vi "generateBarPosAreaCirc.vi"(7 "Number of Denfenders\nWhithout Duelist":i32, 8 "error in (no error)":errorcluster, 9 "AI Parameters":T1={"GotoKick"={"Dist do cone a frente"=150.0, "attacker farback"=1500.0, "Perto"=300.0, "min dist to kick"=150.0, "kick eps"=0.0, "Time to transition"=0.05}, "Attacker"={"CC chute"=0.09, "CC passe"=0.045, "Kick Force"=100.0, "ball-robot Kick"=200.0, "ball-robot Pass"=0.3, "drible\nAttk"=FALSE}, "Defender"={"D max"=1700.0, "Vel p/ robô av"=1000.0, "Kick Force"=100.0, "D atk-def"=0.0, "D farback"=0.0, "drible\ndef"=FALSE, "drible\ngoalie"=FALSE}, "Timeout"={"Field/v in x"=6.0, "Dist Robots"=300, "Dist up in y"=300}, "Pose Striker"={"dist"=200.0, "Numeric"=-4.0, "dist 2"=200.0, "drible\nstriker"=FALSE}, "Dist Stop"=300.0, "D ball out"=200, "D central gap "=150.0, "T pass"=0.0, "Force ++"=0.0, "range kick"=0.0, "Chute alto"=TRUE, "Marcador novo"=TRUE, "drible"=FALSE, "D drible"=300.0, "Versão Striker"=enum."Auto", "Defesa"=enum."ManMark", "Marcador"=enum."Marcar Segundo mais perigoso", "Receptor passe"=enum."Auto", "Área"=enum."Quadrada", "Decisão\nsimples?"=FALSE} {"D drible" format="%#_13g"; "D central gap" format="%#_13g"; "Dist Stop" format="%#_13g"; "Pose Striker"."Numeric" format="%#_13g"; "Defender"."Kick Force" format="%#_13g"; "Defender"."Vel p/ robô av" format="%#_13g"; "Attacker"."ball-robot Kick" format="%#_13g"; "Attacker"."Kick Force" format="%#_13g"; "Attacker"."CC passe" format="%#_13g"; "Attacker"."CC chute" format="%#_13g"; "GotoKick"."kick eps" format="%#_13g"; "GotoKick"."min dist to kick" format="%#_13g"; "GotoKick"."Perto" format="%#_13g"; "GotoKick"."attacker farback" format="%#_13g"; "GotoKick"."Dist do cone a frente" format="%#_13g"}, 10 "Game":refnum<class "Game.lvclass">, 11 "Utilities in":refnum<class "Utilities.lvclass">) -> (0 "error out":errorcluster, 1 "Posição dos Defensores":dbl[][](array[numeric]), 2 "Game out":refnum<class "Game.lvclass">, 3 "Utilities out":refnum<class "Utilities.lvclass">)   [LabVIEW 2023, in "Utilities.lvclass"]
uses:
  Utilities.lvclass
  Vision_class/Old vision/Controls/AI Parameters.ctl
  Game_class/Game.lvclass
  Referee_class/command_interpreted.ctl
  Game_class/Game.lvclass/Game.ctl
  Object_class/Object.lvclass/Object.ctl
  Referee_class/Referee.lvclass/Referee.ctl
  Events_class/Events.lvclass/Events.ctl
  Game_class/Read FieldRef.vi
  Game_class/Read BallRef.vi
  Game_class/Read Referee.vi
  Game_class/Read EventsRef.vi
  Events_class/Read ball_out.vi
  Events_class/Read ball_out_of_vision.vi
  Referee_class/Read command_interpreted.vi
  Object_class/Read x.vi
  Object_class/Read y.vi
  Ball_class/Ball.lvclass
  C:/Users/roboi/Downloads/VSS_AI-Larc2023/Object_class/Object.lvclass
  Field_class/Field.lvclass
  Referee_class/Referee.lvclass
  Events_class/Events.lvclass
panel:
  in  "Array":dbl[][](array[numeric])=[[99999.0, 99999.0], [99999.0, 99999.0], [99999.0, 99999.0], [99999.0, 99999.0], [99999.0, 99999.0], [99999.0, 99999.0], [99999.0, 99999.0]]
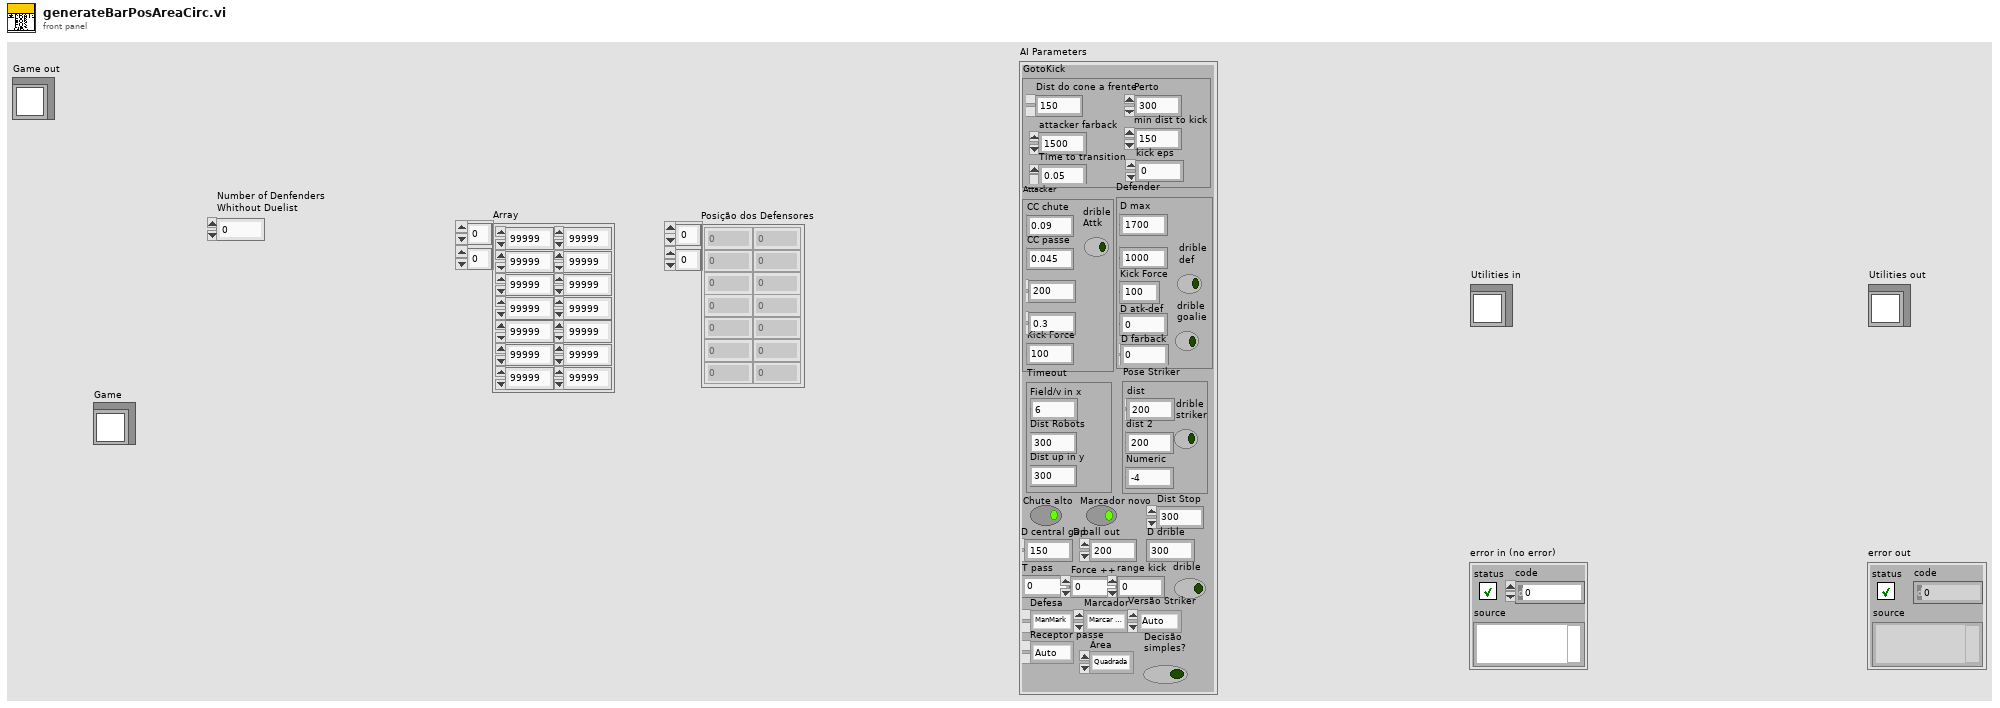
[diagram p1: front panel]
types:
  T1 = typedef "AI Parameters.ctl" = cluster{"GotoKick":cluster{"Dist do cone a frente":dbl, "attacker farback":dbl, "Perto":dbl, "min dist to kick":dbl, "kick eps":dbl, "Time to transition":dbl}, "Attacker":cluster{"CC chute":dbl, "CC passe":dbl, "Kick Force":dbl, "ball-robot Kick":dbl, "ball-robot Pass":dbl, "drible\nAttk":bool}, "Defender":cluster{"D max":dbl, "Vel p/ robô av":dbl, "Kick Force":dbl, "D atk-def":dbl, "D farback":dbl, "drible\ndef":bool, "drible\ngoalie":bool}, "Timeout":cluster{"Field/v in x":dbl, "Dist Robots":u32, "Dist up in y":u32}, "Pose Striker":cluster{"dist":dbl, "Numeric":dbl, "dist 2":dbl, "drible\nstriker":bool}, "Dist Stop":dbl, "D ball out":i32, "D central gap ":dbl, "T pass":dbl, "Force ++":dbl, "range kick":dbl, "Chute alto":bool, "Marcador novo":bool, "drible":bool, "D drible":dbl, "Versão Striker":enum16{"Auto", "3", "2", "1"}, "Defesa":enum16{"ManMark", "Barreira"}, "Marcador":enum16{"Marcar Segundo mais perigoso", "Marcar o mais perigoso"}, "Receptor passe":enum16{"Auto", "2nd Striker", "Striker"}, "Área":enum16{"Quadrada", "Circular"}, "Decisão\nsimples?":bool}
  T2 = typedef "command_interpreted.ctl" = enum16{"Goal Ally", "Goal Enemy", "Ball Placement Enemy", "Ball Placement Ally", "Normal Half Time", "Extra Time  Break", "Extra Half Time", "None", "Post Game", "PKA Normal Start", "Prepare Kickoff Ally", "PKE Normal Start", "Prepare Kickoff Enemy", "Force Start", "Halt", "Timeout", "Prepare Penalty Ally", "Prepare Penalty Enemy", "PPA NormalStart", "PPE Normal Start", "Indirect Free Ally", "Direct Free Enemy", "Direct Free Ally", "Indirect Free Enemy", "Stop"}
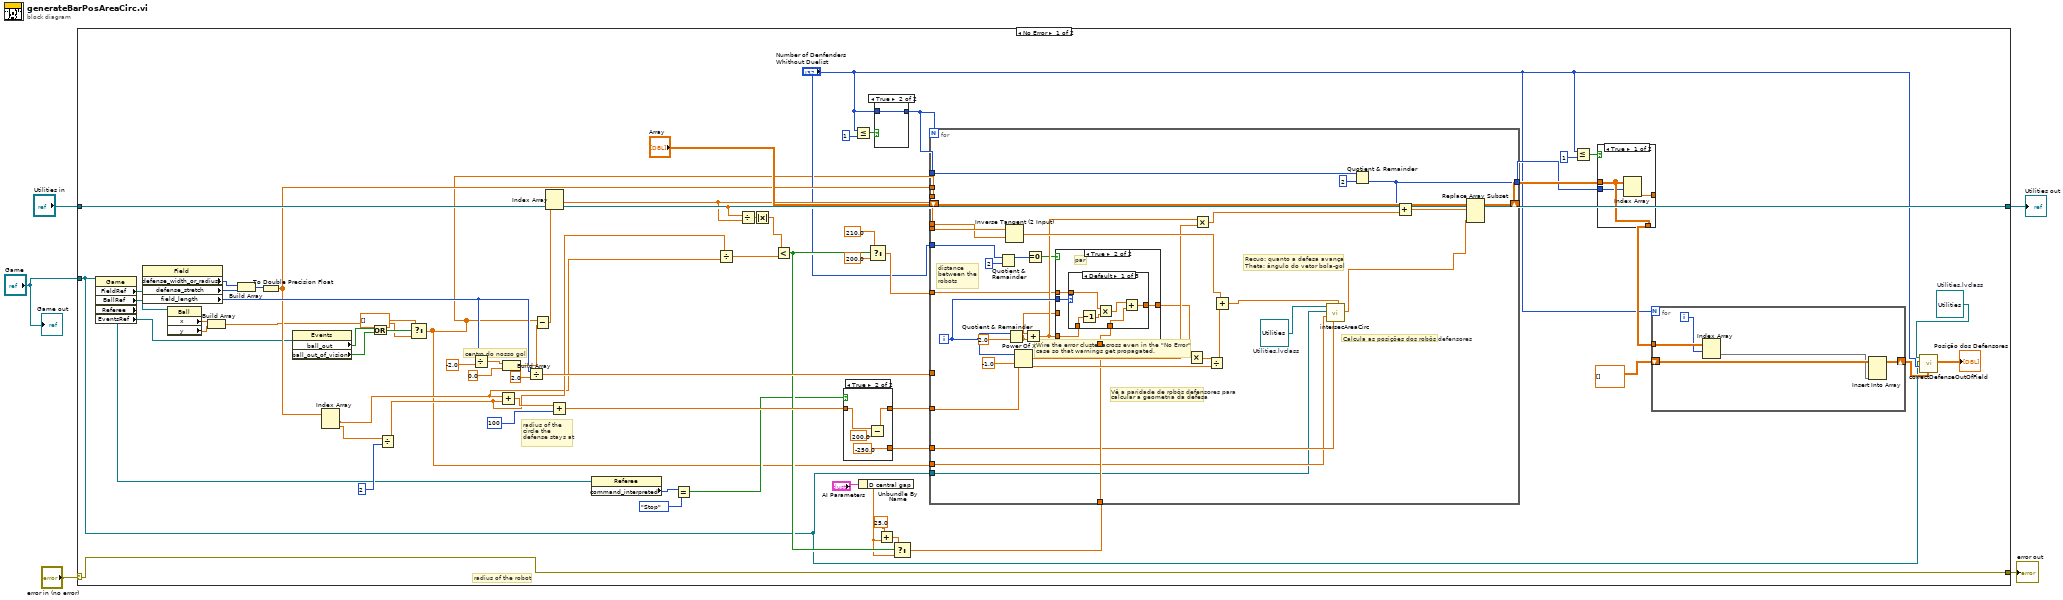
[diagram p0: block diagram]
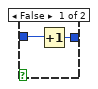
[diagram p2: hidden frame]
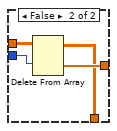
[diagram p3: hidden frame]
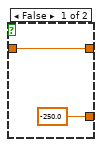
[diagram p4: hidden frame]
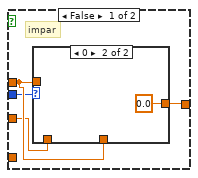
[diagram p5: hidden frame]
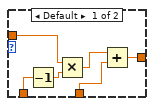
[diagram p6: hidden frame]
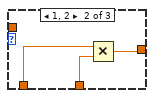
[diagram p7: hidden frame]
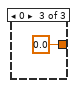
[diagram p8: hidden frame]
diagram:
  n1 = case shown="No Error" "error in (no error)" {
    selector: "error in (no error)" -> [w71 w154]
    tunnel: [w71 w154] -> w4
    tunnel: [w72 w153] -> w2
    tunnel: "Utilities in" -> [w72 w153]
    tunnel: "Game" -> [w6 _]
    frame No Error {
      w30 = refnum<class "Utilities.lvclass"> refnum  # Utilities.lvclass
      # "radius of the circle the defense stays at"
      # "centro do nosso gol"
      # "radius of the robot"
      # "Wire the error cluster across even in the \"No Error\"\ncase so that warnings get propagated."
      n2 = property class="Game"(reference=w6) -> ("FieldRef"=w26:refnum<class "Field.lvclass">, "BallRef"=w29:refnum<class "Ball.lvclass">, "Referee"=w23:refnum<class "Referee.lvclass">, "EventsRef"=w13:refnum<class "Events.lvclass">)  [unwired: 1 in, 2 out]
      n3 = property class="Field"(reference=w26) -> ("defense_width_or_radius"=w18:i32, "defense_stretch"=w25:i32, "field_length"=w19:i32)  [unwired: 1 in, 2 out]
      n4 = property class="Ball"(reference=w29) -> ("x"=w28:dbl, "y"=w27:dbl)  [unwired: 1 in, 2 out]
      n5 = Build Array(w28, w27) -> (w9:dbl[])
      n6 = Build Array(w18, w25) -> (w24:i32[])
      n7 = To Double Precision Float(number=w24) -> (double precision float=w15:dbl[])
      n8 = property class="Events"(reference=w13) -> ("ball_out"=w12:bool, "ball_out_of_vision"=w11:bool)  [unwired: 1 in, 2 out]
      n9 = Index Array(array=w15) -> (element #1=w17:dbl, element #2=w16:dbl)  [unwired: 2 in]
      n10 = Or(x=w12, y=w11) -> (x .or. y?=w10:bool)
      n11 = Divide(x=w16, y=u32 2) -> (x/y=w48:dbl)
      n12 = Select(t=dbl[] [], s=w10, f=w9) -> (s? t:f=w7:dbl[])
      n13 = Divide(x=w19, y=-2.0) -> (x/y=w68:dbl)
      n14 = Add(x=w17, y=w48) -> (x+y=w70:dbl)
      n15 = Build Array(w68, 0.0 ("element")) -> (w49:dbl[])
      n16 = Divide(x=w19, y=2.0) -> (x/y=w63:dbl)
      n17 = Subtract(x=w7, y=w49) -> (x-y=w62:dbl[])
      n18 = Index Array(array=w62) -> (element #1=w46:dbl, element #2=w47:dbl)  [unwired: 2 in]
      n19 = Add(x=w70, y=u32 100) -> (x+y=w61:dbl)
      n20 = property class="Referee"(reference=w23) -> ("command_interpreted"=w22:T2)  [unwired: 1 in, 2 out]
      n21 = Equal?(x=w22, y=command_interpreted."Stop") -> (x = y?=w20:bool)
      n22 = Divide(x=w48, y=w17) -> (x/y=w43:dbl)
      n23 = Divide(x=w47, y=w46) -> (x/y=w45:dbl)
      n24 = Absolute Value(x=w45) -> (abs(x)=w44:dbl)
      n25 = Less?(x=w44, y=w43) -> (x < y?=w39:bool)
      n26 = case shown="True" w20 {
        tunnel: w61 -> [w89 w93]
        tunnel: [w89 w92] -> w60
        tunnel: [-250.0 -250.0] -> w50
        frame False {
        }
        frame True {
          n27 = Subtract(x=w93, y=200.0) -> (x-y=w92:dbl)
        }
      }
      n28 = Less Or Equal?(x="Number of Denfenders\nWhithout Duelist", y=1) -> (x <= y?=w51:bool)
      n29 = Unbundle By Name("AI Parameters") -> ("D central gap"=w36:dbl)
      n30 = Select(t=210.0, s=w39, f=200.0) -> (s? t:f=w40:dbl)
      n31 = case shown="True" w51 {
        tunnel: "Number of Denfenders\nWhithout Duelist" -> [w74 w75]
        tunnel: [w73 w75] -> w55
        frame False {
          n32 = Increment(x=w74) -> (x+1=w73:i32)
        }
        frame True {
        }
      }
      n33 = Add(x=25.0, y=w36) -> (x+y=w34:dbl)
      n34 = Select(t=w34, s=w39, f=w36) -> (s? t:f=w38:dbl)
      n35 = for {
        N: w55 -> [_]
        tunnel: w47 -> [w126]
        tunnel: w46 -> [w125]
        tunnel: w60 -> [w119]
        shift-right: [w115] -> w58
        shift-left: "Array" -> [w114]
        tunnel: w63 -> [_]
        tunnel: [w109] -> w57
        tunnel: w55 -> [w108]
        tunnel: w38 -> [w104]
        tunnel: w7 -> [_]
        tunnel: w15 -> [_]
        tunnel: w50 -> [w103]
        tunnel: w40 -> [w102]
        tunnel: "Number of Denfenders\nWhithout Duelist" -> [w101]
        tunnel: w7 -> [w95]
        tunnel: w6 -> [w94]
        i -> [w107]
        w96 = refnum<class "Utilities.lvclass"> refnum  # Utilities.lvclass
        # "Recuo: quanto a defesa avança\nTheta: ângulo do vetor bola-gol"
        # "Calcula as posições dos robôs defensores"
        # "Vê a paridade de robôs defensores para\ncalcular a geometria da defesa"
        # "distance between the robots"
        n36 = Quotient & Remainder(x=w101, y=2) -> (x-y*floor(x/y)=w99:i32)  [unwired: 1 out]
        n37 = Inverse Tangent (2 Input)(1:w125, 2:w126) -> (0:w122:dbl)
        n38 = Quotient & Remainder(x=w107, y=2.0) -> (x-y*floor(x/y)=w117:dbl, floor(x/y)=w97:dbl)
        n39 = Power Of X(1:-1.0, 2:w107) -> (0:w113:dbl)
        n40 = Add(x=w117, y=w97) -> (x+y=w106:dbl)
        n41 = Equal To 0?(x=w99) -> (x = 0?=w98:bool)
        n42 = case shown="True" w98 {
          tunnel: w107 -> [w128 w142]
          tunnel: w106 -> [_ w141]
          tunnel: [w129 w140] -> w105
          tunnel: w104 -> [_ w139]
          tunnel: w102 -> [w130 w138]
          tunnel: w97 -> [w127 _]
          frame False {
            # "impar"
            n43 = case shown="0" w128 {
              tunnel: [w134 0.0 ("x")] -> w129
              tunnel: w127 -> [w136 _]
              tunnel: w130 -> [w132 _]
              tunnel: w130 -> [w131 _]
              frame Default {
                n44 = Decrement(x=w136) -> (x-1=w135:dbl)
                n45 = Multiply(x=w131, y=w135) -> (x*y=w133:dbl)
                n46 = Add(x=w133, y=w132) -> (x+y=w134:dbl)
              }
              frame 0 {
              }
            }
          }
          frame True {
            # "par"
            n47 = case shown="Default" w142 {
              tunnel: [w146 w149 0.0 ("x")] -> w140
              tunnel: w141 -> [w148 w151 _]
              tunnel: w139 -> [w144 w150 _]
              tunnel: w138 -> [w143 _ _]
              frame Default {
                n48 = Decrement(x=w148) -> (x-1=w147:dbl)
                n49 = Multiply(x=w143, y=w147) -> (x*y=w145:dbl)
                n50 = Add(x=w145, y=w144) -> (x+y=w146:dbl)
              }
              frame 1, 2 {
                n51 = Multiply(x=w151, y=w150) -> (x*y=w149:dbl)
              }
              frame 0 {
              }
            }
          }
        }
        n52 = Multiply(x=w105, y=w113) -> (x*y=w123:dbl)
        n53 = Multiply(x=w106, y=w113) -> (x*y=w111:dbl)
        n54 = Divide(x=w123, y=w119) -> (x/y=w121:dbl)
        n55 = Add(x=w122, y=w121) -> (x+y=w120:dbl)
        n56 = call "intersecAreaCirc.vi"("theta"=w120, "Recuo"=w103, "Ball/Enemy\nPosition"=w95, "Game"=w94, "Utilities in"=w96) -> ("Position"=w116:dbl[])  [unwired: 4 in, 2 out]
        n57 = Quotient & Remainder(x=w108, y=2) -> (floor(x/y)=w109:i32)  [unwired: 1 out]
        n58 = Add(x=w109, y=w111) -> (x+y=w112:dbl)
        n59 = Replace Array Subset(array=w114, new element=w116, index (row)=w112) -> (w115:dbl[][])  [unwired: 1 in]
      }
      n60 = Less Or Equal?(x="Number of Denfenders\nWhithout Duelist", y=1) -> (x <= y?=w54:bool)
      n61 = case shown="True" w54 {
        tunnel: [w78 w82] -> _
        tunnel: w58 -> [w77 w81]
        tunnel: w57 -> [w76 w80]
        tunnel: [w77 w79] -> w56
        frame True {
          n62 = Index Array(array=w77, index (row)=w76) -> (element=w78:dbl[])  [unwired: 1 in]
        }
        frame False {
          n63 = Delete From Array(array=w81, index (row)=w80) -> (deleted portion=w82:dbl[], array with subset deleted=w79:dbl[][])  [unwired: 2 in]
        }
      }
      n64 = for {
        N: "Number of Denfenders\nWhithout Duelist" -> [_]
        shift-right: [w86] -> w31
        shift-left: dbl[][] [] ("Array 2") -> [w87]
        tunnel: w56 -> [w85]
        i -> [w84]
        n65 = Index Array(array=w85, index (row)=w84) -> (element=w83:dbl[])  [unwired: 1 in]
        n66 = Insert Into Array(array=w87, new element=w83) -> (w86:dbl[][])  [unwired: 2 in]
      }
      n67 = call "correctDefenseOutOfField.vi"("Pos Centers Back in"=w31, "Number of Defenders\nWithout Duelist"="Number of Denfenders\nWhithout Duelist", "Game"=w6, "Utilities in"=w30) -> ("Pos Centers Back out"=→"Posição dos Defensores":dbl[][])  [unwired: 5 in, 2 out]
    }
    frame Error {
    }
  }
  "error out" <- w4
  "Utilities out" <- w2
  "Game out" <- "Game"
